vi "CU_stopClassifier.vi"(8 "error in (no error)":errorcluster, 11 "ClassifierClass in":refnum<class "ClassifierClass.lvclass">) -> (0 "error out":errorcluster, 3 "ClassifierClass out":refnum<class "ClassifierClass.lvclass">)   [LabVIEW 2016, in "Classifier.lvlib" / "ClassifierClass.lvclass"]
uses:
  ClassifierClass.lvclass
  ClassifierClass.lvclass/ClassifierClass.ctl
  <vilib>/xml/Close Reference(Node).vi
  <vilib>/xml/NI_XML.lvlib
panel:
  # "This VI is a part of BCI Design library, http://www.ru-bci.org \nCopyright © 2020, Sotnikov Peter, All rights reserved. License: GNU GPLv3"
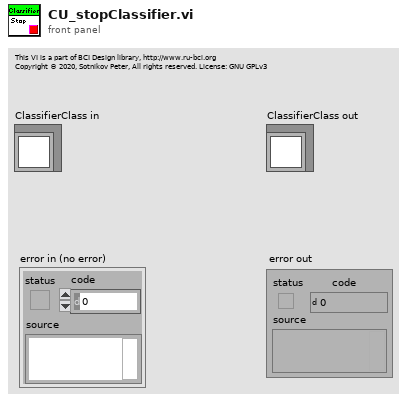
[diagram p1: front panel]
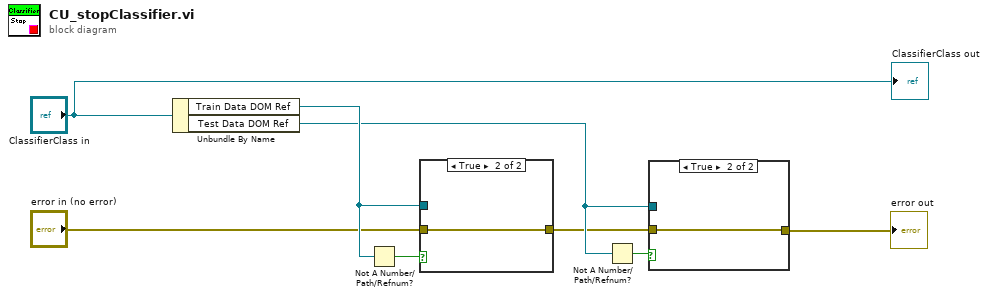
[diagram p0: block diagram]
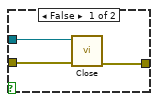
[diagram p2: hidden frame]
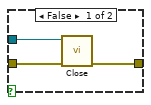
[diagram p3: hidden frame]
diagram:
  n1 = Unbundle By Name("ClassifierClass in") -> ("Train Data DOM Ref"=w7:refnum<k20>, "Test Data DOM Ref"=w3:refnum<k20>)
  n2 = Not A Number/Path/Refnum?(number/path/refnum=w7) -> (NaN/Path/Refnum?=w6:bool)
  n3 = case shown="True" w6 {
    tunnel: w7 -> [w11 _]
    tunnel: "error in (no error)" -> [w10 w12]
    tunnel: [w9 w12] -> w2
    frame False {
      n4 = call-poly <vilib>:"Close.vi"("error in (no error)"=w10, "node"=w11) -> ("error out"=w9:errorcluster)  [unwired: 7 in]
    }
    frame True {
    }
  }
  n5 = Not A Number/Path/Refnum?(number/path/refnum=w3) -> (NaN/Path/Refnum?=w4:bool)
  n6 = case shown="True" w4 {
    tunnel: w3 -> [w15 _]
    tunnel: w2 -> [w14 w16]
    tunnel: [w13 w16] -> w1
    frame False {
      n7 = call-poly <vilib>:"Close.vi"("error in (no error)"=w14, "node"=w15) -> ("error out"=w13:errorcluster)  [unwired: 7 in]
    }
    frame True {
    }
  }
  "error out" <- w1
  "ClassifierClass out" <- "ClassifierClass in"
